vi "Z6_Beamline.PC Remote Controlled.vi"(0 "i ref in":refnum<vi>, 2 "Remote Controller":string="N/A", 5 "error in (no error)":errorcluster) -> (14 "i ref out":refnum<vi>, 19 "error out":errorcluster)   [LabVIEW 2009]
doc: "This VI enables or disables GUI elements."
uses:
  Z6_Beamline.lvlib
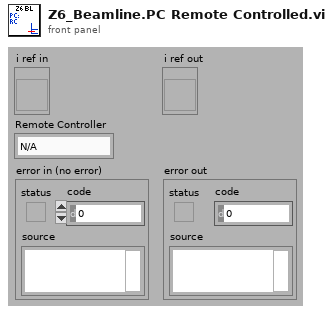
[diagram p1: front panel]
types:
  T1 = typedef "Z6_Beamline.lvlib/Z6_Beamline.i attribute.ctl" = cluster{"GUI Refs":cluster{"Northtower ok":refnum<vi>, "Southtower ok":refnum<vi>, "Frontends ok":refnum<vi>, "100TW COS ok":refnum<vi>}, "Refs BL Northtower":refnum<vi>[], "Refs BL Southtower":refnum<vi>[], "Refs BL 100TW COS":refnum<vi>[], "Color State PHELIX":cluster{"Service Name":string, "State":i16}, "State Subsystems":cluster{"Northtower":bool, "Southtower":bool, "Frontends":bool, "100TW COS":bool}}
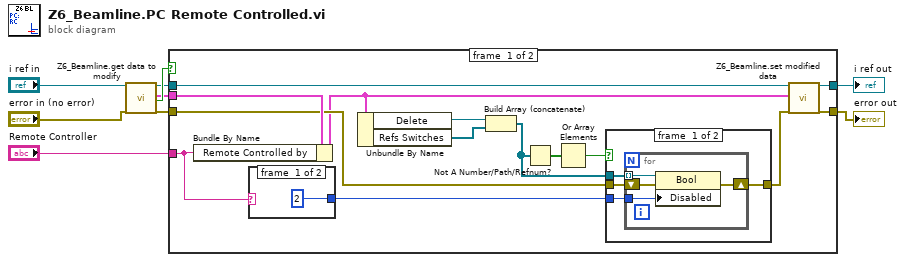
[diagram p0: block diagram]
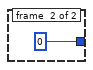
[diagram p2: hidden frame]
diagram:
  n1 = call "Z6_Beamline.get data to modify.vi"("i ref in"="i ref in", "error in (no error)"="error in (no error)") -> ("i ref out"=w3:refnum<vi>, "i attribute"=w7:T1, "timed out"=w8:bool, "error out"=w5:errorcluster)  [unwired: 14 in]
  n2 = case shown="False" w8 {
    tunnel: w3 -> [w23 w36]
    tunnel: [w22 w36] -> w4
    tunnel: w5 -> [w19 w35]
    tunnel: [w21 w35] -> w6
    tunnel: w7 -> [w20 _]
    tunnel: "Remote Controller" -> [w12 _]
    frame #0 {
      n3 = Bundle By Name(cluster=w20, "Remote Controlled by"=w12) -> (w17:T1)
      n4 = case shown="Default" w12 {
        tunnel: [u8 2 ("Disabled") u8 0 ("Disabled")] -> w11
        frame #0 {
        }
        frame #1 {
        }
      }
      n5 = Unbundle By Name(w17) -> ("Delete"=w16:refnum<vi>, "Refs Switches"=w10:refnum<vi>[])
      n6 = Build Array (concatenate)(w16, w10) -> (w15:refnum<vi>[])
      n7 = Not A Number/Path/Refnum?(number/path/refnum=w15) -> (NaN/Path/Refnum?=w14:bool[])
      n8 = Or Array Elements(Boolean array=w14) -> (logical OR=w13:bool)
      n9 = case shown="False" w13 {
        tunnel: w19 -> [w29 w34]
        tunnel: [w28 w34] -> w18
        tunnel: w15 -> [w27 _]
        tunnel: w11 -> [w26 _]
        frame #0 {
          n10 = for {
            tunnel: w27 -> [w31] mode=indexing
            shift-right: [w32] -> w28
            shift-left: w29 -> [w33]
            tunnel: w26 -> [w30]
            n11 = property class="Bool"(reference=w31, error in=w33, "Disabled"=w30) -> (error out=w32:errorcluster)  [unwired: 1 out]
          }
        }
        frame #1 {
        }
      }
      n12 = call "Z6_Beamline.set modified data.vi"("i ref in"=w23, "i attribute"=w17, "error in (no error)"=w18) -> ("i ref out"=w22:refnum<vi>, "error out"=w21:errorcluster)  [unwired: 15 in]
    }
    frame #1 {
    }
  }
  "error out" <- w6
  "i ref out" <- w4
